vi "usb get libusb version string.vi"(10 "dest_buffer_length":u32, 11 "dest":string) -> (2 "function return":i32, 3 "dest out":string)   [LabVIEW 2019, in "apdm.lvlib"]
doc: "APDM_EXPORT int apdm_usb_get_libusb_version_string(char *dest, const uint32_t dest_buffer_length);"
uses:
  apdm.lvlib
  Lee Lab/CP FES Walking 2018/Code/Working/LabVIEW/apdm.dll
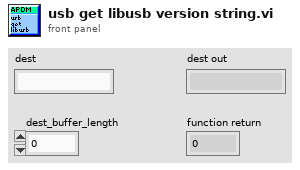
[diagram p1: front panel]
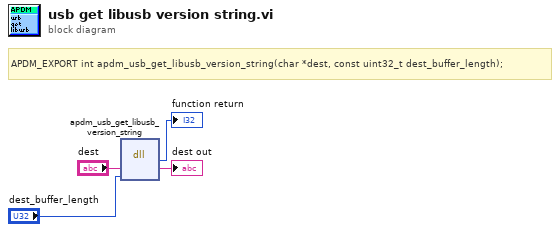
[diagram p0: block diagram]
diagram:
  # "APDM_EXPORT int apdm_usb_get_libusb_version_string(char *dest, const uint32_t dest_buffer_length);"
  n1 = dll-call lib="C:/Users/jfalesi/Dropbox/Lee Lab/CP FES Walking 2018/Code/Working/LabVIEW/apdm.*" fn="apdm_usb_get_libusb_version_string"("dest"="dest", "dest_buffer_length"="dest_buffer_length") -> (→"function return":i32, "dest"=→"dest out":string)  [unwired: 4 in, 2 out]
